vi "GetTargetName.vi"(8 "error in (no error)":errorcluster, 11 "VIA in":refnum<class "BotSpeak.lvclass">) -> (0 "error out":errorcluster, 2 "TargetName":string, 3 "VIA out":refnum<class "BotSpeak.lvclass">)   [LabVIEW 2012, in "BotSpeak.lvclass"]
uses:
  <userlib>/botspeak/VIs/BotSpeak.lvclass
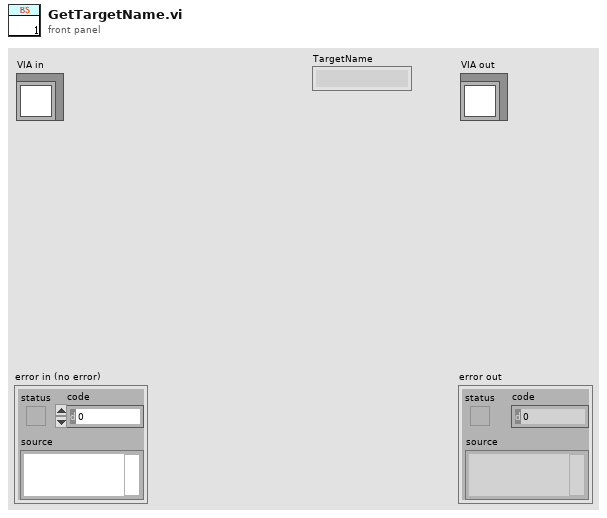
[diagram p1: front panel]
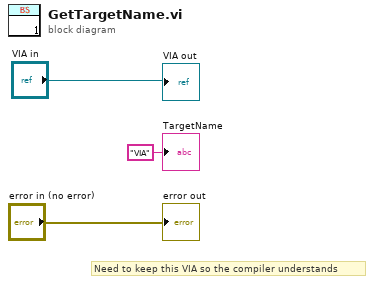
[diagram p0: block diagram]
diagram:
  # "Need to keep this VIA so the compiler understands"
  "error out" <- "error in (no error)"
  "VIA out" <- "VIA in"
  "TargetName" <- "VIA" ("TargetName")
